vi "test-SwerveModuleState.vi"(8 "error in (no error)":errorcluster) -> (0 "error out":errorcluster, 3 "ALL TESTS PASSED":bool)   [LabVIEW 2019]
uses:
  <vilib>/Rock Robotics/WPI/ThirdParty/JAS_Junk/TrajLib/SWERVE_DRIVE_MODULE_STATE.ctl
  <vilib>/Rock Robotics/WPI/ThirdParty/JAS_Junk/TrajLib/ROTATION2D.ctl
  <vilib>/Rock Robotics/WPI/ThirdParty/JAS_Junk/TrajLib/Rotation_Minus.vi
  <vilib>/Rock Robotics/WPI/ThirdParty/JAS_Junk/TrajLib/Rotation_GetRadians.vi
  <vilib>/Rock Robotics/WPI/ThirdParty/JAS_Junk/TrajLib/Rotation_RotateBy.vi
  <vilib>/Rock Robotics/WPI/ThirdParty/JAS_Junk/TrajLib/Rotation_UnaryMinus.vi
  <vilib>/Rock Robotics/WPI/ThirdParty/JAS_Junk/TrajLib/Rotation_CreateXY.vi
  <vilib>/Rock Robotics/WPI/ThirdParty/JAS_Junk/TrajLib/Util_CalcDist.vi
  <vilib>/Rock Robotics/WPI/ThirdParty/JAS_Junk/TrajLib/Trajectory_Library.lvlib
panel:
  out "Test 1B":bool
  out "T1B":T1={"Speed"=0.0, "Angle"={"VALUE"=0.0, "COS"=1.0, "SIN"=0.0}} {"Angle"."SIN" format="%13.4f"; "Angle"."COS" format="%13.4f"; "Angle"."VALUE" format="%13.4f"}
  out "Test 1A":bool
  out "T1A":T1={"Speed"=0.0, "Angle"={"VALUE"=0.0, "COS"=1.0, "SIN"=0.0}} {"Angle"."SIN" format="%13.4f"; "Angle"."COS" format="%13.4f"; "Angle"."VALUE" format="%13.4f"}
  out "Test 0B":bool
  out "T0B":T1={"Speed"=0.0, "Angle"={"VALUE"=0.0, "COS"=1.0, "SIN"=0.0}} {"Angle"."SIN" format="%13.4f"; "Angle"."COS" format="%13.4f"; "Angle"."VALUE" format="%13.4f"}
  out "Test 0A":bool
  out "T91 Ang = reversed":T1={"Speed"=0.0, "Angle"={"VALUE"=0.0, "COS"=1.0, "SIN"=0.0}} {"Angle"."SIN" format="%13.4f"; "Angle"."COS" format="%13.4f"; "Angle"."VALUE" format="%13.4f"}
  out "T90  Ang = small":T1={"Speed"=0.0, "Angle"={"VALUE"=0.0, "COS"=1.0, "SIN"=0.0}} {"Angle"."SIN" format="%13.4f"; "Angle"."COS" format="%13.4f"; "Angle"."VALUE" format="%13.4f"}
  out "T3":T1={"Speed"=0.0, "Angle"={"VALUE"=0.0, "COS"=1.0, "SIN"=0.0}} {"Angle"."SIN" format="%13.4f"; "Angle"."COS" format="%13.4f"; "Angle"."VALUE" format="%13.4f"}
  out "T2":T1={"Speed"=0.0, "Angle"={"VALUE"=0.0, "COS"=1.0, "SIN"=0.0}} {"Angle"."SIN" format="%13.4f"; "Angle"."COS" format="%13.4f"; "Angle"."VALUE" format="%13.4f"}
  out "T1":i32
  out "T0A":T1={"Speed"=0.0, "Angle"={"VALUE"=0.0, "COS"=1.0, "SIN"=0.0}} {"Angle"."SIN" format="%13.4f"; "Angle"."COS" format="%13.4f"; "Angle"."VALUE" format="%13.4f"}
  # "SwerveModuleState Test"
  # "THESE ARE OLD TESTS..."
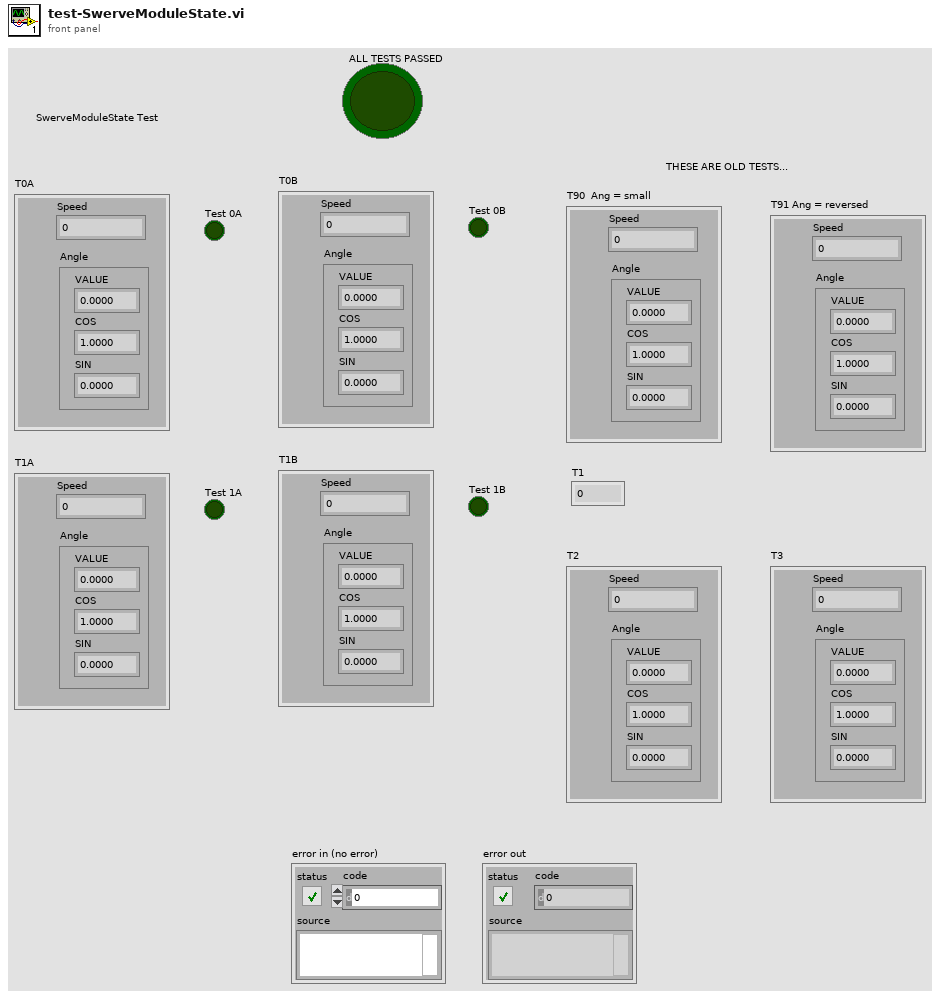
[diagram p1: front panel]
types:
  T1 = typedef "Trajectory_Library.lvlib/SWERVE_DRIVE_MODULE_STATE.ctl" = cluster{"Speed":dbl, "Angle":T2}
  T2 = typedef "Trajectory_Library.lvlib/ROTATION2D.ctl" = cluster{"VALUE":dbl, "COS":dbl, "SIN":dbl}
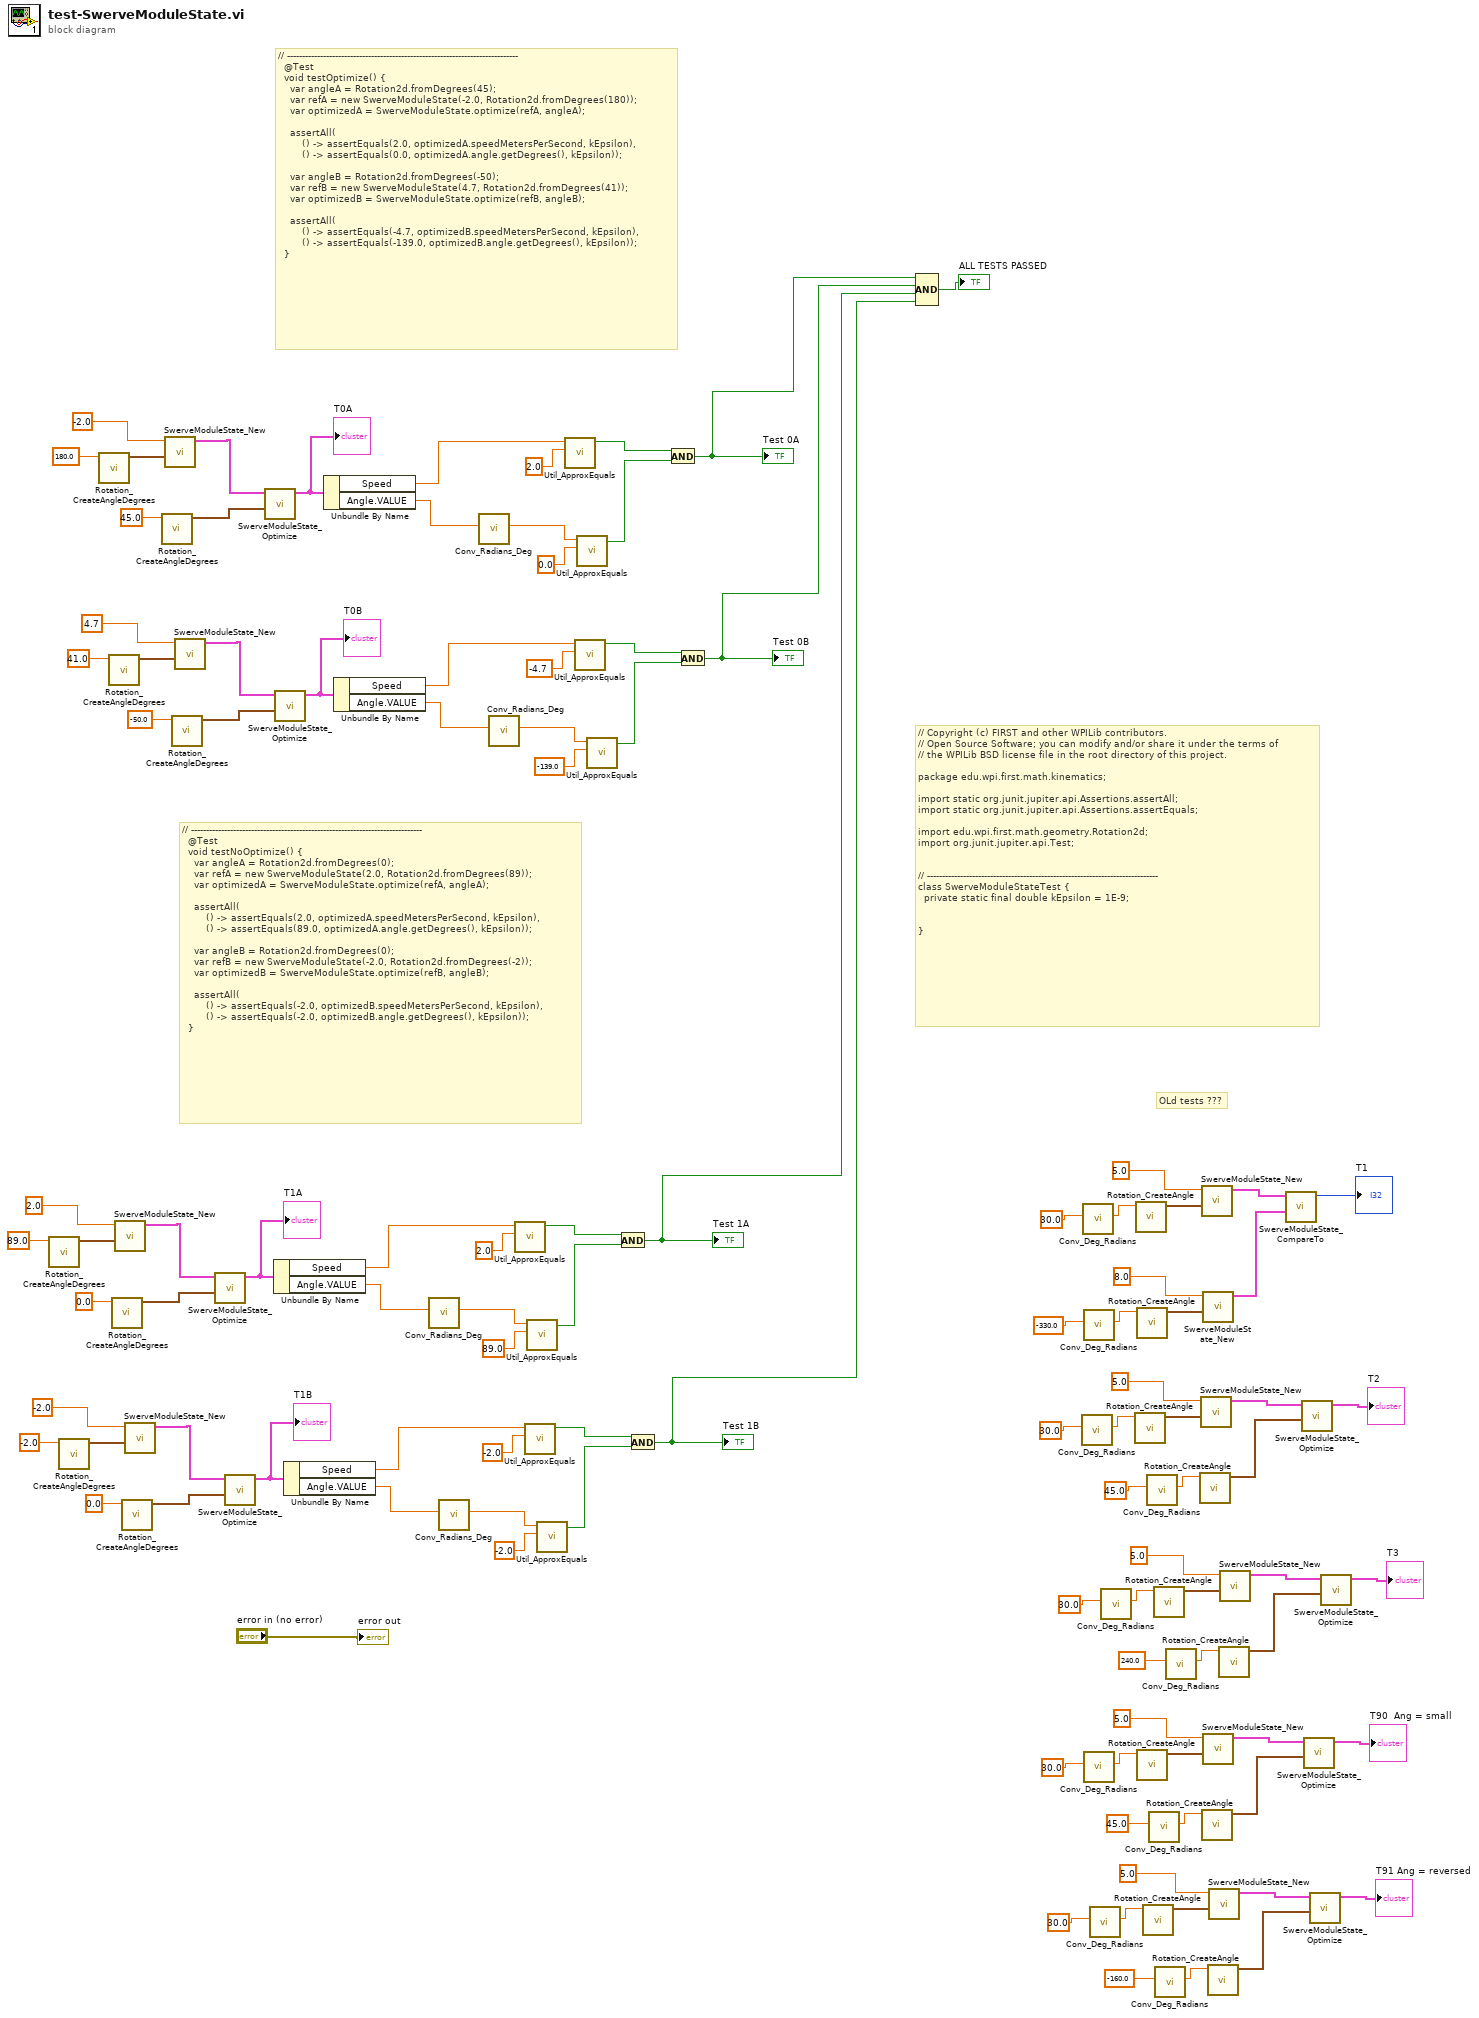
[diagram p0: block diagram]
diagram:
  # "OLd tests ???"
  # "// -----------------------------------------------------------------------------\n  @Test\n  void testNoOptimize() {\n    var angleA = Rotation2d.fromDegrees(0);\n    var refA = new SwerveModuleState(2.0, Rotation2d.fromDegrees(89));\n    var optimizedA = SwerveModuleState.optimize(refA, angleA);\n\n    assertAll(\n        () -> assertEquals(2.0, optimizedA.speedMetersPerSecond, kEpsilon),\n        () -> assertEquals(89.0, optimizedA.angle.getDegrees(), kEpsilon));\n\n    var angleB = Rotation2d.fromDegrees(0);\n    var refB = new SwerveModuleState(-2.0, Rotation2d.fromDegrees(-2));\n    var optimizedB = SwerveModuleState.optimize(refB, angleB);\n\n    assertAll(\n        () -> assertEquals(-2.0, optimizedB.speedMetersPerSecond, kEpsilon),\n        () -> assertEquals(-2.0, optimizedB.angle.getDegrees(), kEpsilon));\n  }"
  # "// -----------------------------------------------------------------------------\n  @Test\n  void testOptimize() {\n    var angleA = Rotation2d.fromDegrees(45);\n    var refA = new SwerveModuleState(-2.0, Rotation2d.fromDegrees(180));\n    var optimizedA = SwerveModuleState.optimize(refA, angleA);\n\n    assertAll(\n        () -> assertEquals(2.0, optimizedA.speedMetersPerSecond, kEpsilon),\n        () -> assertEquals(0.0, optimizedA.angle.getDegrees(), kEpsilon));\n\n    var angleB = Rotation2d.fromDegrees(-50);\n    var refB = new SwerveModuleState(4.7, Rotation2d.fromDegrees(41));\n    var optimizedB = SwerveModuleState.optimize(refB, angleB);\n\n    assertAll(\n        () -> assertEquals(-4.7, optimizedB.speedMetersPerSecond, kEpsilon),\n        () -> assertEquals(-139.0, optimizedB.angle.getDegrees(), kEpsilon));\n  }"
  # "// Copyright (c) FIRST and other WPILib contributors.\n// Open Source Software; you can modify and/or share it under the terms of\n// the WPILib BSD license file in the root directory of this project.\n\npackage edu.wpi.first.math.kinematics;\n\nimport static org.junit.jupiter.api.Assertions.assertAll;\nimport static org.junit.jupiter.api.Assertions.assertEquals;\n\nimport edu.wpi.first.math.geometry.Rotation2d;\nimport org.junit.jupiter.api.Test;\n\n\n// -----------------------------------------------------------------------------\nclass SwerveModuleStateTest {\n  private static final double kEpsilon = 1E-9;\n\n\n}"
  n1 = call <vilib>:"Rotation_CreateAngleDegrees.vi"("Angle_Degrees"=89.0 ("y")) -> ("ROTATION"=w30:T2)  [unwired: 10 in]
  n2 = call <vilib>:"Rotation_CreateAngleDegrees.vi"("Angle_Degrees"=-2.0 ("y")) -> ("ROTATION"=w16:T2)  [unwired: 10 in]
  n3 = call <vilib>:"Rotation_CreateAngleDegrees.vi"("Angle_Degrees"=180.0 ("y")) -> ("ROTATION"=w108:T2)  [unwired: 10 in]
  n4 = call <vilib>:"Rotation_CreateAngleDegrees.vi"("Angle_Degrees"=41.0 ("y")) -> ("ROTATION"=w46:T2)  [unwired: 10 in]
  n5 = call <vilib>:"Rotation_CreateAngleDegrees.vi"("Angle_Degrees"=0.0 ("y")) -> ("ROTATION"=w26:T2)  [unwired: 10 in]
  n6 = call <vilib>:"SwerveModuleState_New.vi"("ROTATION"=w30, "Speed"=2.0) -> ("SWERVE_DRIVE_MODULE_STATE"=w27:T1)  [unwired: 9 in]
  n7 = call <vilib>:"Rotation_CreateAngleDegrees.vi"("Angle_Degrees"=0.0 ("y")) -> ("ROTATION"=w12:T2)  [unwired: 10 in]
  n8 = call <vilib>:"SwerveModuleState_New.vi"("ROTATION"=w16, "Speed"=-2.0) -> ("SWERVE_DRIVE_MODULE_STATE"=w13:T1)  [unwired: 9 in]
  n9 = call <vilib>:"Rotation_CreateAngleDegrees.vi"("Angle_Degrees"=45.0 ("y")) -> ("ROTATION"=w57:T2)  [unwired: 10 in]
  n10 = call <vilib>:"SwerveModuleState_New.vi"("ROTATION"=w108, "Speed"=-2.0) -> ("SWERVE_DRIVE_MODULE_STATE"=w58:T1)  [unwired: 9 in]
  n11 = call <vilib>:"Rotation_CreateAngleDegrees.vi"("Angle_Degrees"=-50.0 ("y")) -> ("ROTATION"=w42:T2)  [unwired: 10 in]
  n12 = call <vilib>:"SwerveModuleState_New.vi"("ROTATION"=w46, "Speed"=4.7) -> ("SWERVE_DRIVE_MODULE_STATE"=w43:T1)  [unwired: 9 in]
  n13 = call <vilib>:"SwerveModuleState_Optimize.vi"("CurrentAngle"=w26, "Desired State"=w27) -> ("out SWERVE_DRIVE_MODULE_STATE"=w20:T1)  [unwired: 9 in]
  "T1A" <- w20
  n14 = call <vilib>:"SwerveModuleState_Optimize.vi"("CurrentAngle"=w12, "Desired State"=w13) -> ("out SWERVE_DRIVE_MODULE_STATE"=w6:T1)  [unwired: 9 in]
  "T1B" <- w6
  n15 = call <vilib>:"SwerveModuleState_Optimize.vi"("CurrentAngle"=w57, "Desired State"=w58) -> ("out SWERVE_DRIVE_MODULE_STATE"=w51:T1)  [unwired: 9 in]
  "T0A" <- w51
  n16 = Unbundle By Name(w20) -> ("Speed"=w21:dbl, "Angle.VALUE"=w25:dbl)
  n17 = call <vilib>:"SwerveModuleState_Optimize.vi"("CurrentAngle"=w42, "Desired State"=w43) -> ("out SWERVE_DRIVE_MODULE_STATE"=w36:T1)  [unwired: 9 in]
  "T0B" <- w36
  n18 = Unbundle By Name(w6) -> ("Speed"=w7:dbl, "Angle.VALUE"=w11:dbl)
  n19 = Unbundle By Name(w51) -> ("Speed"=w52:dbl, "Angle.VALUE"=w56:dbl)
  n20 = Unbundle By Name(w36) -> ("Speed"=w37:dbl, "Angle.VALUE"=w41:dbl)
  n21 = call <vilib>:"Conv_Radians_Deg.vi"("Radians"=w25) -> ("Degrees"=w22:dbl)  [unwired: 10 in]
  n22 = call <vilib>:"Conv_Radians_Deg.vi"("Radians"=w11) -> ("Degrees"=w8:dbl)  [unwired: 10 in]
  n23 = call <vilib>:"Conv_Radians_Deg.vi"("Radians"=w56) -> ("Degrees"=w53:dbl)  [unwired: 10 in]
  n24 = call <vilib>:"Conv_Radians_Deg.vi"("Radians"=w41) -> ("Degrees"=w38:dbl)  [unwired: 10 in]
  n25 = call <vilib>:"Util_ApproxEquals.vi"("Value 2"=2.0, "Value 1"=w21) -> ("ApproxEquals"=w19:bool)  [unwired: 9 in]
  n26 = call <vilib>:"Util_ApproxEquals.vi"("Value 2"=-2.0, "Value 1"=w7) -> ("ApproxEquals"=w5:bool)  [unwired: 9 in]
  n27 = call <vilib>:"Util_ApproxEquals.vi"("Value 2"=89.0, "Value 1"=w22) -> ("ApproxEquals"=w18:bool)  [unwired: 9 in]
  n28 = call <vilib>:"Util_ApproxEquals.vi"("Value 2"=-2.0, "Value 1"=w8) -> ("ApproxEquals"=w4:bool)  [unwired: 9 in]
  n29 = call <vilib>:"Util_ApproxEquals.vi"("Value 2"=2.0, "Value 1"=w52) -> ("ApproxEquals"=w50:bool)  [unwired: 9 in]
  n30 = call <vilib>:"Util_ApproxEquals.vi"("Value 2"=-4.7, "Value 1"=w37) -> ("ApproxEquals"=w35:bool)  [unwired: 9 in]
  n31 = call <vilib>:"Util_ApproxEquals.vi"("Value 2"=0.0, "Value 1"=w53) -> ("ApproxEquals"=w49:bool)  [unwired: 9 in]
  n32 = call <vilib>:"Util_ApproxEquals.vi"("Value 2"=-139.0, "Value 1"=w38) -> ("ApproxEquals"=w34:bool)  [unwired: 9 in]
  n33 = And(x=w19, y=w18) -> (x .and. y?=w3:bool)
  "Test 1A" <- w3
  n34 = And(x=w5, y=w4) -> (x .and. y?=w2:bool)
  "Test 1B" <- w2
  n35 = And(x=w50, y=w49) -> (x .and. y?=w48:bool)
  "Test 0A" <- w48
  n36 = And(x=w35, y=w34) -> (x .and. y?=w33:bool)
  "Test 0B" <- w33
  n37 = Compound Arithmetic op=AND(w48, w33, w3, w2) -> (→"ALL TESTS PASSED":bool)
  n38 = call <vilib>:"Conv_Deg_Radians.vi"("Degress"=30.0 ("y")) -> ("Radians"=w96:dbl)  [unwired: 10 in]
  n39 = call <vilib>:"Conv_Deg_Radians.vi"("Degress"=30.0 ("y")) -> ("Radians"=w107:dbl)  [unwired: 10 in]
  n40 = call <vilib>:"Conv_Deg_Radians.vi"("Degress"=-330.0 ("y")) -> ("Radians"=w103:dbl)  [unwired: 10 in]
  n41 = call <vilib>:"Conv_Deg_Radians.vi"("Degress"=30.0 ("y")) -> ("Radians"=w78:dbl)  [unwired: 10 in]
  n42 = call <vilib>:"Conv_Deg_Radians.vi"("Degress"=30.0 ("y")) -> ("Radians"=w69:dbl)  [unwired: 10 in]
  n43 = call <vilib>:"Conv_Deg_Radians.vi"("Degress"=30.0 ("y")) -> ("Radians"=w87:dbl)  [unwired: 10 in]
  n44 = call <vilib>:"Rotation_CreateAngle.vi"("Angle"=w96) -> ("ROTATION"=w93:T2)  [unwired: 10 in]
  n45 = call <vilib>:"Rotation_CreateAngle.vi"("Angle"=w107) -> ("ROTATION"=w104:T2)  [unwired: 10 in]
  n46 = call <vilib>:"Rotation_CreateAngle.vi"("Angle"=w103) -> ("ROTATION"=w100:T2)  [unwired: 10 in]
  n47 = call <vilib>:"Rotation_CreateAngle.vi"("Angle"=w78) -> ("ROTATION"=w76:T2)  [unwired: 10 in]
  n48 = call <vilib>:"Rotation_CreateAngle.vi"("Angle"=w69) -> ("ROTATION"=w67:T2)  [unwired: 10 in]
  n49 = call <vilib>:"Conv_Deg_Radians.vi"("Degress"=45.0 ("y")) -> ("Radians"=w90:dbl)  [unwired: 10 in]
  n50 = call <vilib>:"Conv_Deg_Radians.vi"("Degress"=45.0 ("y")) -> ("Radians"=w73:dbl)  [unwired: 10 in]
  n51 = call <vilib>:"Rotation_CreateAngle.vi"("Angle"=w87) -> ("ROTATION"=w85:T2)  [unwired: 10 in]
  n52 = call <vilib>:"Conv_Deg_Radians.vi"("Degress"=-160.0 ("y")) -> ("Radians"=w64:dbl)  [unwired: 10 in]
  n53 = call <vilib>:"Conv_Deg_Radians.vi"("Degress"=240.0 ("y")) -> ("Radians"=w82:dbl)  [unwired: 10 in]
  n54 = call <vilib>:"Rotation_CreateAngle.vi"("Angle"=w90) -> ("ROTATION"=w88:T2)  [unwired: 10 in]
  n55 = call <vilib>:"SwerveModuleState_New.vi"("ROTATION"=w93, "Speed"=5.0) -> ("SWERVE_DRIVE_MODULE_STATE"=w92:T1)  [unwired: 9 in]
  n56 = call <vilib>:"SwerveModuleState_New.vi"("ROTATION"=w104, "Speed"=5.0) -> ("SWERVE_DRIVE_MODULE_STATE"=w98:T1)  [unwired: 9 in]
  n57 = call <vilib>:"Rotation_CreateAngle.vi"("Angle"=w73) -> ("ROTATION"=w71:T2)  [unwired: 10 in]
  n58 = call <vilib>:"SwerveModuleState_New.vi"("ROTATION"=w100, "Speed"=8.0) -> ("SWERVE_DRIVE_MODULE_STATE"=w97:T1)  [unwired: 9 in]
  n59 = call <vilib>:"SwerveModuleState_New.vi"("ROTATION"=w76, "Speed"=5.0) -> ("SWERVE_DRIVE_MODULE_STATE"=w75:T1)  [unwired: 9 in]
  n60 = call <vilib>:"Rotation_CreateAngle.vi"("Angle"=w64) -> ("ROTATION"=w62:T2)  [unwired: 10 in]
  n61 = call <vilib>:"SwerveModuleState_New.vi"("ROTATION"=w67, "Speed"=5.0) -> ("SWERVE_DRIVE_MODULE_STATE"=w66:T1)  [unwired: 9 in]
  n62 = call <vilib>:"Rotation_CreateAngle.vi"("Angle"=w82) -> ("ROTATION"=w80:T2)  [unwired: 10 in]
  n63 = call <vilib>:"SwerveModuleState_New.vi"("ROTATION"=w85, "Speed"=5.0) -> ("SWERVE_DRIVE_MODULE_STATE"=w84:T1)  [unwired: 9 in]
  n64 = call <vilib>:"SwerveModuleState_CompareTo.vi"("other SWERVE_DRIVE_MODULE_STATE"=w97, "in SWERVE_DRIVE_MODULE_STATE"=w98) -> ("Compare"=→"T1":i32)  [unwired: 9 in]
  n65 = call <vilib>:"SwerveModuleState_Optimize.vi"("CurrentAngle"=w88, "Desired State"=w92) -> ("out SWERVE_DRIVE_MODULE_STATE"=→"T2":T1)  [unwired: 9 in]
  n66 = call <vilib>:"SwerveModuleState_Optimize.vi"("CurrentAngle"=w71, "Desired State"=w75) -> ("out SWERVE_DRIVE_MODULE_STATE"=→"T90  Ang = small":T1)  [unwired: 9 in]
  n67 = call <vilib>:"SwerveModuleState_Optimize.vi"("CurrentAngle"=w62, "Desired State"=w66) -> ("out SWERVE_DRIVE_MODULE_STATE"=→"T91 Ang = reversed":T1)  [unwired: 9 in]
  n68 = call <vilib>:"SwerveModuleState_Optimize.vi"("CurrentAngle"=w80, "Desired State"=w84) -> ("out SWERVE_DRIVE_MODULE_STATE"=→"T3":T1)  [unwired: 9 in]
  "error out" <- "error in (no error)"
